vi "z bytes copy from slice.vi"(8 "error in (no error)":errorcluster, 10 "slice":cluster{}, 11 "this_":cluster{}) -> (0 "error out":errorcluster, 3 "this_ out":cluster{})   [LabVIEW 2021, in "zenohc.lvlib"]
doc: "void z_bytes_copy_from_slice(struct z_owned_bytes_t *this_,\n const struct z_loaned_slice_t *slice);"
uses:
  zenohc.lvlib
  zenohc.dll
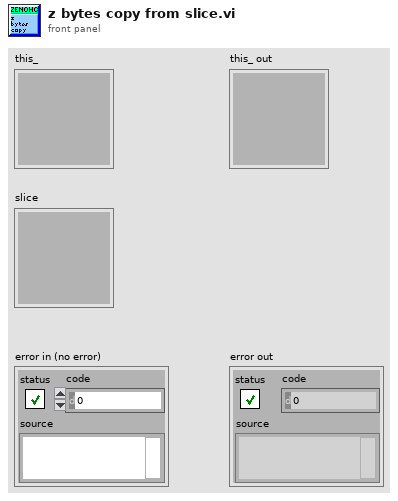
[diagram p1: front panel]
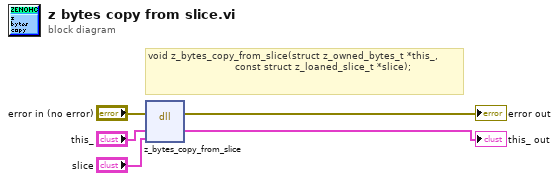
[diagram p0: block diagram]
diagram:
  # "void z_bytes_copy_from_slice(struct z_owned_bytes_t *this_,\n                             const struct z_loaned_slice_t *slice);"
  n1 = dll-call lib="D:/dev/zenoh_labview/zenohc/zenohc.*" fn="z_bytes_copy_from_slice"(error in="error in (no error)", "this_"="this_", "slice"="slice") -> (error out=→"error out":errorcluster, "this_"=→"this_ out":cluster{})  [unwired: 4 in, 1 out]
